vi "Auswerten.vi"(8 "LIN Ausgabetabelle":refnum<vi>, 9 "Komponente:":refnum<vi>, 10 "max. Flow Weighted Mean:":refnum<vi>) -> (0 "Konzentration Komponente":dbl, 1 "Komponente:":T1, 2 "max. Flow Weighted Mean:":T1, 3 "Konzentration FlowWeightedMean":dbl, 4 "Limit in ppm":dbl, 5 "[%]":dbl)   [LabVIEW 2020, in "EPA 1065.lvlib" / "Interference verificaton 1065-366.lvlib"]
uses:
  Interference verificaton 1065-366.lvlib
  Visualisierungs Elemente/String - Ausgabefeld.ctl
  <vilib>/Utility/miscctls.llb/LVRowAndColumnTypeDef.ctl
  Sprachverwaltung/FGV Aktion Tabelle zerlegen.ctl
  Aktion FGV Interference.ctl
  Sprachverwaltung/Sprachverwaltung.lvlib
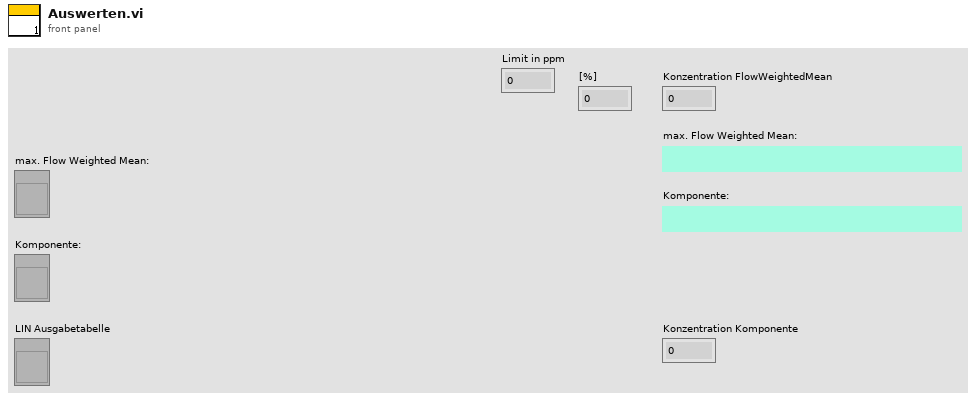
[diagram p1: front panel]
types:
  T1 = typedef "String - Ausgabefeld.ctl" = string
  T2 = typedef "EPA 1065.lvlib/Interference verificaton 1065-366.lvlib/Aktion FGV Interference.ctl" = enum16{"Lesen", "TestKonfig", "TestSetting", "Einheiten", "Ergebnis", "Laden", "Tabelle", "Speichern", "löschen"}
  T3 = typedef "Sprachverwaltung.lvlib/FGV Aktion Tabelle zerlegen.ctl" = enum16{"laden", "vereinzeln", "speichern"}
  T4 = typedef "LVRowAndColumnTypeDef.ctl" = cluster{"Row":i32, "Column":i32}
  T5 = typedef "EPA 1065.lvlib/Interference verificaton 1065-366.lvlib/TestKonfig.ctl" = cluster{"CH4:":u16, "Ethane:":u16, "NMHC:":u16, "NMNEHC:":u16, "Komp 1 aktiv:":bool, "Komp 2 aktiv:":bool, "Komp 3 aktiv:":bool, "Komp 4 aktiv:":bool, "Modus":T6, "CG Aufschaltzeit:":dbl, "Interferent 1: CO2":u16, "Interferent 2: H2O":u16, "Interferent 3: CH4":u16, "Interferent 4: C2H6 / C3H8":u16, "Gasflaschen Nr.:":string, "Gasflaschen Nr.: 3":string, "Gasflaschen Nr.: 4":string, "Inter 1 aktiv":bool, "Inter 2 aktiv":bool, "Inter 3 aktiv":bool, "Inter 4 aktiv":bool, "Accuracy":string, "Accuracy 3":string, "Accuracy 4":string, "Konzentration 1:":dbl, "Konzentration 2:":dbl, "Konzentration 3:":dbl, "Konzentration 4:":dbl, "Flow weighted mean 1:":dbl, "Flow weighted mean 2:":dbl, "Flow weighted mean 3:":dbl, "Flow weighted mean 4:":dbl}
  T6 = typedef "EPA 1065.lvlib/Interference verificaton 1065-366.lvlib/Modus.ctl" = u16
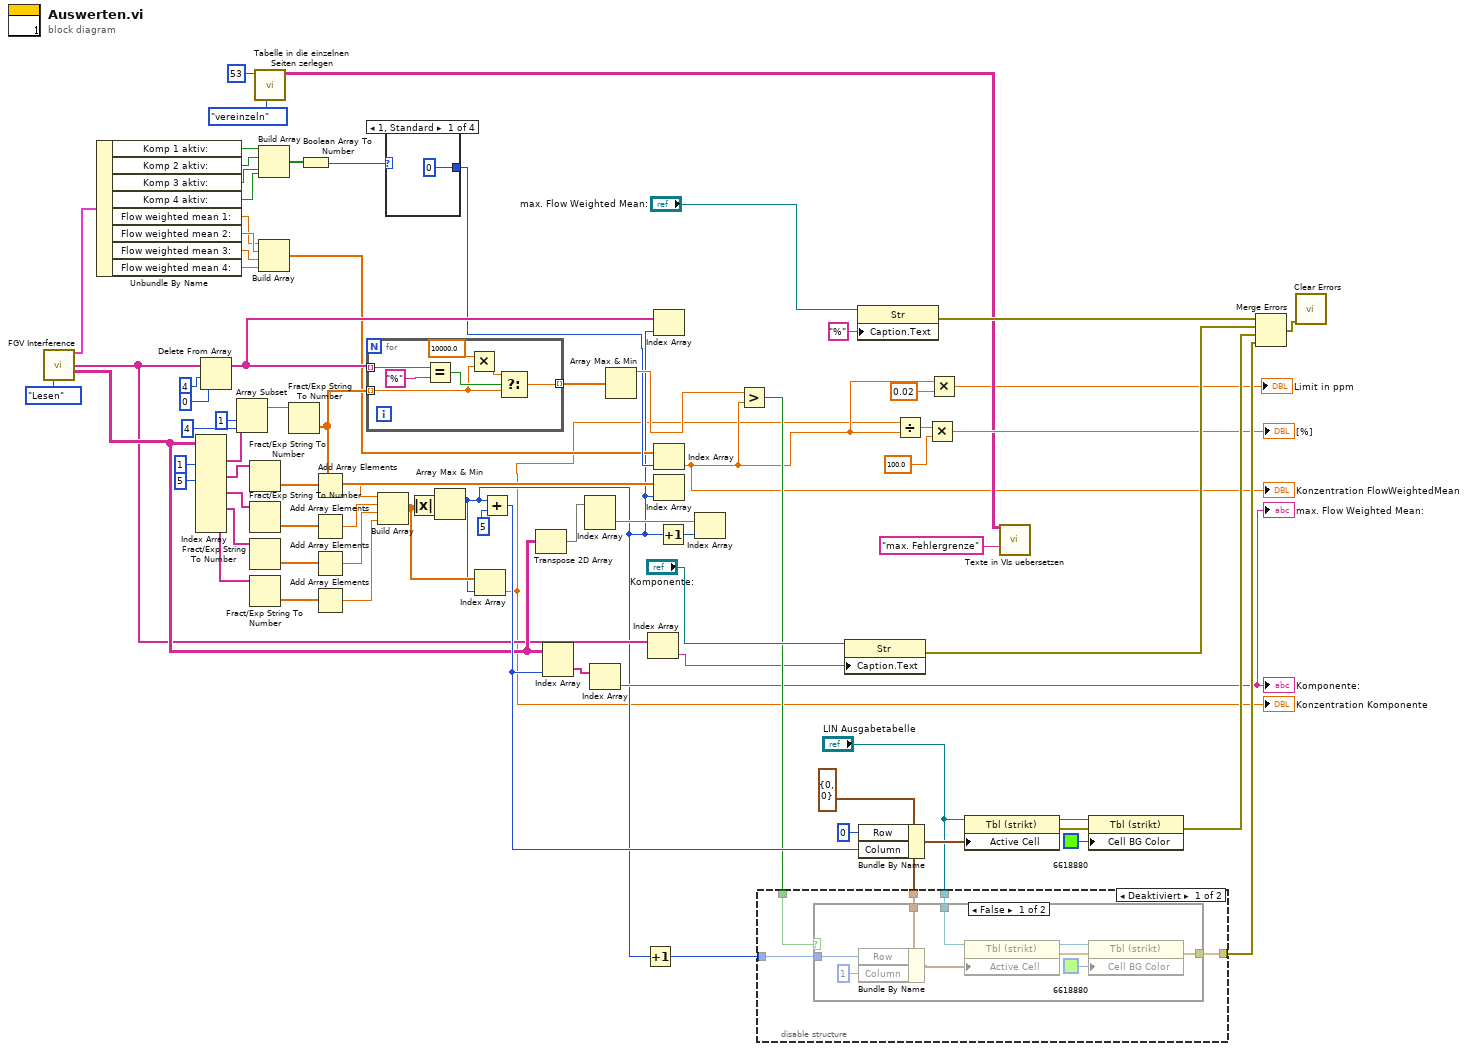
[diagram p0: block diagram]
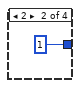
[diagram p2: hidden frame]
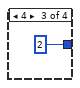
[diagram p3: hidden frame]
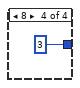
[diagram p4: hidden frame]
diagram:
  w73 = T4 {"Row"=0, "Column"=0} ("Aktive Zelle:Aktive Zelle")
  n1 = call "FGV Interference.vi"("Aktion FGV Interference"=Aktion_FGV_Interference."Lesen") -> ("TestKonfig"=w28:T5, "Êinheiten"=w12:string[], "Tabelle"=w29:T1[][])  [unwired: 9 in, 3 out]
  n2 = Unbundle By Name(w28) -> ("Komp 1 aktiv:"=w27:bool, "Komp 2 aktiv:"=w26:bool, "Komp 3 aktiv:"=w25:bool, "Komp 4 aktiv:"=w24:bool, "Flow weighted mean 1:"=w17:dbl, "Flow weighted mean 2:"=w18:dbl, "Flow weighted mean 3:"=w19:dbl, "Flow weighted mean 4:"=w20:dbl)
  n3 = Index Array(array=w29, index (col) #1=1 ("Deaktivierter Index (Spalte)"), index (col) #2=5 ("Index (Spalte)")) -> (element #1=w50:T1[], element #2=w51:T1[], element #3=w52:T1[], element #4=w53:T1[], element #5=w6:T1[])  [unwired: 8 in]
  n4 = Delete From Array(array=w12, length=4 ("Länge"), index=0 ("Index")) -> (array with subset deleted=w54:string[])  [unwired: 1 out]
  n5 = Array Subset(array=w50, index=1 ("Index"), length=4 ("Länge")) -> (w46:T1[])
  n6 = Fract/Exp String To Number(string=w51) -> (number=w10:dbl[])  [unwired: 3 in, 1 out]
  n7 = Fract/Exp String To Number(string=w52) -> (number=w9:dbl[])  [unwired: 3 in, 1 out]
  n8 = Fract/Exp String To Number(string=w53) -> (number=w8:dbl[])  [unwired: 3 in, 1 out]
  n9 = Fract/Exp String To Number(string=w6) -> (number=w7:dbl[])  [unwired: 3 in, 1 out]
  n10 = call "Tabelle in die einzelnen Seiten zerlegen.vi"("Aktion"=FGV_Aktion_Tabelle_zerlegen."vereinzeln", "Index (Seite)"=53) -> ("Sprachliste"=w37:string[][])  [unwired: 7 in, 2 out]
  n11 = Build Array(w27, w26, w25, w24) -> (w23:bool[])
  n12 = Build Array(w17, w18, w19, w20) -> (w16:dbl[])
  n13 = Fract/Exp String To Number(string=w46) -> (number=w59:dbl[])  [unwired: 3 in, 1 out]
  n14 = Boolean Array To Number(Boolean array=w23) -> (number=w22:u32)
  n15 = Add Array Elements(numeric array=w10) -> (sum=w55:dbl)
  n16 = Add Array Elements(numeric array=w9) -> (sum=w56:dbl)
  n17 = Add Array Elements(numeric array=w8) -> (sum=w57:dbl)
  n18 = Add Array Elements(numeric array=w7) -> (sum=w5:dbl)
  n19 = for {
    tunnel: w54 -> [w82] mode=indexing
    tunnel: w59 -> [w81] mode=indexing
    tunnel: [w80] -> w11 mode=indexing
    n20 = Equal?(x=w82, y="%") -> (x = y?=w85:bool)
    n21 = Multiply(x=10000.0, y=w81) -> (x*y=w84:dbl)
    n22 = Select(t=w84, s=w85, f=w81) -> (s? t:f=w80:dbl)
  }
  n23 = Build Array(w55, w56, w57, w5) -> (w4:dbl[])
  n24 = case shown="1, Standard" w22 {
    tunnel: [0 1 2 3] -> w21
    frame 1, Default {
    }
    frame 2 {
    }
    frame 4 {
    }
    frame 8 {
    }
  }
  n25 = Absolute Value(x=w4) -> (abs(x)=w3:dbl[])
  n26 = Array Max & Min(array=w3) -> (max index (indices)=w2:i32)  [unwired: 3 out]
  n27 = Index Array(array=w4, index=w2) -> (element=w1:dbl)
  "Konzentration Komponente" <- w1
  n28 = Add(x=w2, y=5) -> (x+y=w71:i32)
  n29 = Transpose 2D Array(2D array=w29) -> (transposed array=w47:T1[][])
  n30 = Index Array(array=w29, index (col)=w71) -> (element=w58:T1[])  [unwired: 1 in]
  n31 = Index Array(array=w47) -> (element=w60:T1[])  [unwired: 2 in]
  n32 = Index Array(array=w58) -> (element=→"max. Flow Weighted Mean:" →"Komponente:":T1)  [unwired: 1 in]
  n33 = Array Max & Min(array=w11) -> (max value=w41:dbl)  [unwired: 3 out]
  n34 = Increment(x=w2) -> (x+1=w43:i32)
  n35 = Index Array(array=w12) -> (element=w36:string)  [unwired: 1 in]
  n36 = Index Array(array=w54, index=w2) -> ()  [unwired: 1 out]
  n37 = Index Array(array=w16, index=w21) -> (element=w15:dbl)
  "Konzentration FlowWeightedMean" <- w15
  n38 = Index Array(array=w59, index=w2) -> ()  [unwired: 1 out]
  n39 = Increment(x=w2) -> (x+1=w42:i32)
  n40 = Index Array(array=w60, index=w42) -> ()  [unwired: 1 out]
  n41 = Greater?(x=w41, y=w15) -> (0:w40:bool)
  n42 = disable-structure shown="Deaktiviert" {
    disable-tunnel: [w95 _] -> w78
    disable-tunnel: w73 -> [w94 _]
    disable-tunnel: "LIN Ausgabetabelle" -> [w93 _]
    disable-tunnel: w43 -> [w92 _]
    disable-tunnel: w40 -> [w91 _]
    frame Disabled {
      n43 = case shown="False" w91 {
        tunnel: [w104 _] -> w95
        tunnel: w94 -> [w101 _]
        tunnel: w93 -> [w99 _]
        tunnel: w92 -> [w96 _]
        frame False {
          n44 = Bundle By Name(cluster=w101, "Row"=w96, "Column"=1) -> (w100:T4)
          n45 = property on="Eigenschaftsknoten" class="Tbl (strikt)"(reference=w99, "Active Cell"=w100) -> (reference out=w103:refnum<vi>, error out=w98:errorcluster)  [unwired: 1 in]
          n46 = property on="Eigenschaftsknoten" class="Tbl (strikt)"(reference=w103, error in=w98, "Cell BG Color"=u32 6618880) -> (error out=w104:errorcluster)  [unwired: 1 out]
        }
        frame True {
        }
      }
    }
    frame Enabled {
    }
  }
  n47 = property on="Eigenschaftsknoten" class="Str"(reference="Komponente:", "Caption.Text"=w36) -> (error out=w76:errorcluster)  [unwired: 1 in, 1 out]
  n48 = property on="Eigenschaftsknoten" class="Str"(reference="max. Flow Weighted Mean:", "Caption.Text"="%" ("Untertitel.Text")) -> (error out=w75:errorcluster)  [unwired: 1 in, 1 out]
  n49 = Bundle By Name(cluster=w73, "Row"=0, "Column"=w71) -> (w79:T4)
  n50 = Divide(x=w1, y=w15) -> (x/y=w34:dbl)
  n51 = Multiply(x=w34, y=100.0) -> (x*y=→"[%]":dbl)
  n52 = Multiply(x=w15, y=0.02) -> (x*y=→"Limit in ppm":dbl)
  n53 = property on="Eigenschaftsknoten" class="Tbl (strikt)"(reference="LIN Ausgabetabelle", "Active Cell"=w79) -> (reference out=w68:refnum<vi>, error out=w67:errorcluster)  [unwired: 1 in]
  n54 = call "Texte in VIs uebersetzen.vi"("Sprachliste"=w37, "String zum Übersetzen"="max. Fehlergrenze" ("String - Ausgabefeld")) -> ()  [unwired: 9 in, 5 out]
  n55 = property on="Eigenschaftsknoten" class="Tbl (strikt)"(reference=w68, error in=w67, "Cell BG Color"=u32 6618880) -> (error out=w77:errorcluster)  [unwired: 1 out]
  n56 = Merge Errors(w75, w76, w77, w78) -> (w74:errorcluster)
  n57 = call <vilib>:"Clear Errors.vi"("error in (no error)"=w74) -> ()  [unwired: 5 in, 2 out]
